vi "Get Clients Info.vi"(8 "error in (no error)":errorcluster, 11 "JKI_Python_Server in":refnum<class "Server.lvclass">) -> (0 "error out":errorcluster, 1 "Number of Connections":u32, 2 "Client Connected":bool, 3 "JKI_Python_Server out":refnum<class "Server.lvclass">, 5 "Connections Info":T1[](array[typedef]))   [LabVIEW 2013, in "JKI_Python_Bridge_for_LV.lvlib" / "Server.lvclass"]
uses:
  Server.lvclass
  <vilib>/addons/_JKI.lib/_jki_lib_tcp_server.llb/TCP Server Public Connections Info Cluster__jki_lib_tcp_server.ctl
  Server.lvclass/Server.ctl
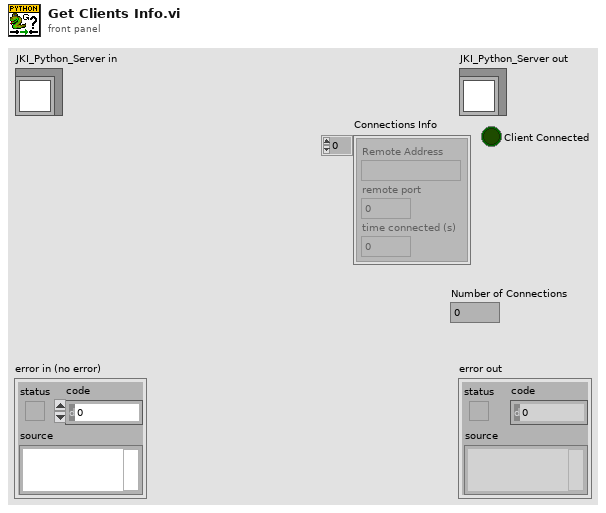
[diagram p1: front panel]
types:
  T1 = typedef "TCP Server Public Connections Info Cluster__jki_lib_tcp_server.ctl" = cluster{"Remote Address":string, "remote port":u16, "time connected (s)":dbl}
  T2 = typedef "JKI_Python_Bridge_for_LV.lvlib/Server.lvclass/Class Private Data - Cluster.ctl" = cluster{"TCP Server RefNum":T3, "TCP port (50007)":u16, "max connections (0: no limit)":u32, "net address (0: Listen on All Adaptors)":u32, "Nodes":T4[], "Public Events":T5}
  T3 = typedef "TCP Server Object RefNum__jki_lib_tcp_server.ctl" = refnum<k1>
  T4 = typedef "JKI_Python_Bridge_for_LV.lvlib/Server.lvclass/Python Node.ctl" = cluster{"Name":string, "Python Method Call":refnum<user-event>, "Call Handle":refnum<class "CallHandler.lvclass">}
  T5 = typedef "JKI_Python_Bridge_for_LV.lvlib/Server.lvclass/Public Events - Cluster.ctl" = cluster{"Stop Nodes":refnum<user-event>}
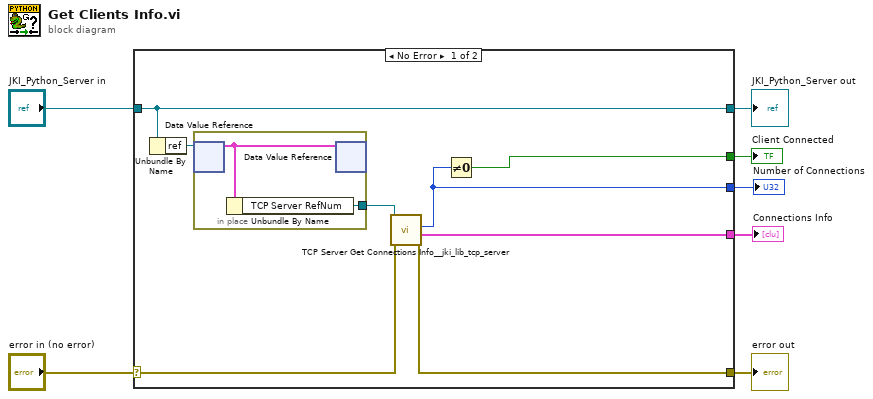
[diagram p0: block diagram]
diagram:
  n1 = case shown="No Error" "error in (no error)" {
    selector: "error in (no error)" -> [w14 w19]
    tunnel: [w13 w19] -> w6
    tunnel: [w15 w18] -> w4
    tunnel: "JKI_Python_Server in" -> [w15 w18]
    tunnel: [w12 _] -> w3
    tunnel: [w11 _] -> w2
    tunnel: [w10 _] -> w1
    frame No Error {
      n2 = Unbundle By Name(w15) -> ("ref"=w9:refnum<data-value>)
      n3 = in-place {
        in-place-border: [w16] -> w8
        n4 = in-place-dvr #1(w9) -> (w17:T2)  [unwired: 1 out]
        n5 = Unbundle By Name(w17) -> ("TCP Server RefNum"=w16:T3)
        n6 = in-place-dvr #1(w17) -> ()  [unwired: 2 out]
      }
      n7 = call <vilib>:"TCP Server Get Connections Info__jki_lib_tcp_server.vi"("error in (no error)"=w14, "Object RefNum"=w8) -> ("error out"=w13:errorcluster, "Connections Info"=w12:T1[], "Number of Connections"=w10:u32)  [unwired: 7 out]
      n8 = Not Equal To 0?(x=w10) -> (x != 0?=w11:bool)
    }
    frame Error {
    }
  }
  "error out" <- w6
  "JKI_Python_Server out" <- w4
  "Connections Info" <- w3
  "Client Connected" <- w2
  "Number of Connections" <- w1
